vi "Build Field Elements.vi"(10 "Field Half Graph":refnum<vi>, 11 "Field Settings":T1={"Exchange Left"=102.0, "Exchange Right"=150.0, "Power Cube Zone Left"=139.5, "Power Cube Zone Right"=139.5, "Switch Left"=85.25, "Switch Right"=85.25, "Switch Front"=140.0, "Switch Back"=196.0, "Platform Left"=95.25, "Platform Right"=95.25, "Platform Front"=261.47, "Slalom Depth"=235.235}) -> (3 "Field Half":cluster{dbl[], dbl[]}[](graph)=[{[0.0, 36.0, 36.0, 0.0, 0.0], [222.0, 222.0, 174.0, 174.0, 222.0]}, {[101.0, 140.0, 140.0, 101.0, 101.0], [184.5, 184.5, 139.5, 139.5, 184.5]}, {[140.0, 196.0, 196.0, 140.0, 140.0], [238.75, 238.75, 85.25, 85.25, 238.75]}, {[196.0, 209.0, 209.0, 196.0, 196.0], [85.25, 85.25, 98.25, 98.25, 85.25]}, {[196.0, 209.0, 209.0, 196.0, 196.0], [113.35, 113.35, 126.35, 126.35, 113.35]}, {[196.0, 209.0, 209.0, 196.0, 196.0], [141.45, 141.45, 154.45, 154.45, 141.45]}, {[196.0, 209.0, 209.0, 196.0, 196.0], [169.55, 169.55, 182.55, 182.55, 169.55]}, {[196.0, 209.0, 209.0, 196.0, 196.0], [197.65, 197.65, 210.65, 210.65, 197.65]}, {[196.0, 209.0, 209.0, 196.0, 196.0], [225.75, 225.75, 238.75, 238.75, 225.75]}, {[261.47, 386.0, 386.0, 261.47, 261.47], [228.75, 228.75, 95.25, 95.25, 228.75]}])   [LabVIEW 2017]
uses:
  Typedef/Field Settings.ctl
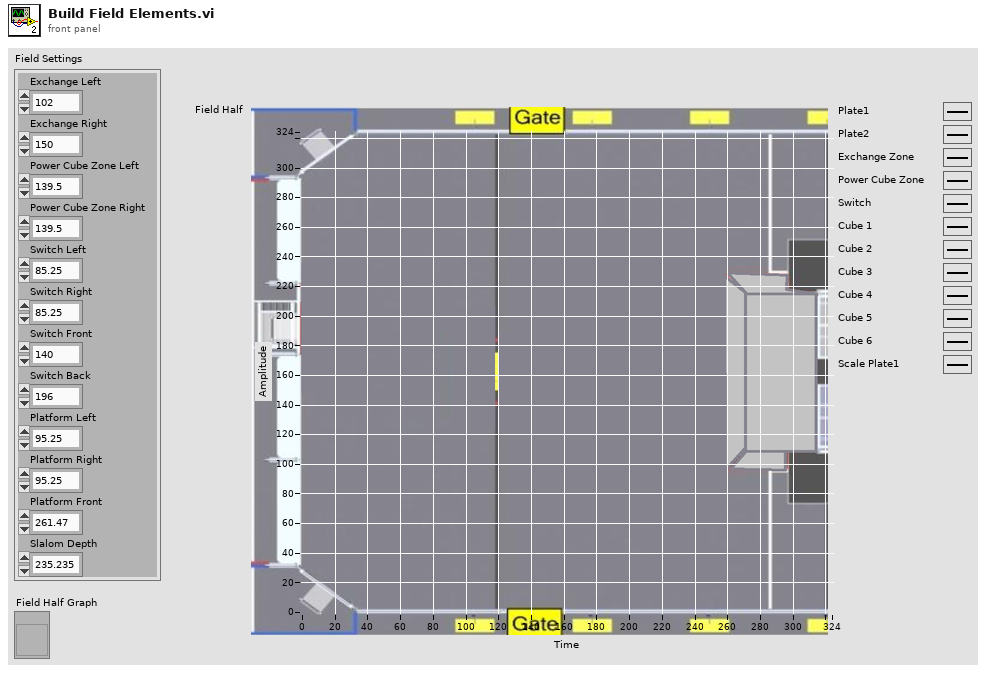
[diagram p1: front panel]
types:
  T1 = typedef "Field Settings.ctl" = cluster{"Exchange Left":dbl, "Exchange Right":dbl, "Power Cube Zone Left":dbl, "Power Cube Zone Right":dbl, "Switch Left":dbl, "Switch Right":dbl, "Switch Front":dbl, "Switch Back":dbl, "Platform Left":dbl, "Platform Right":dbl, "Platform Front":dbl, "Slalom Depth":dbl}
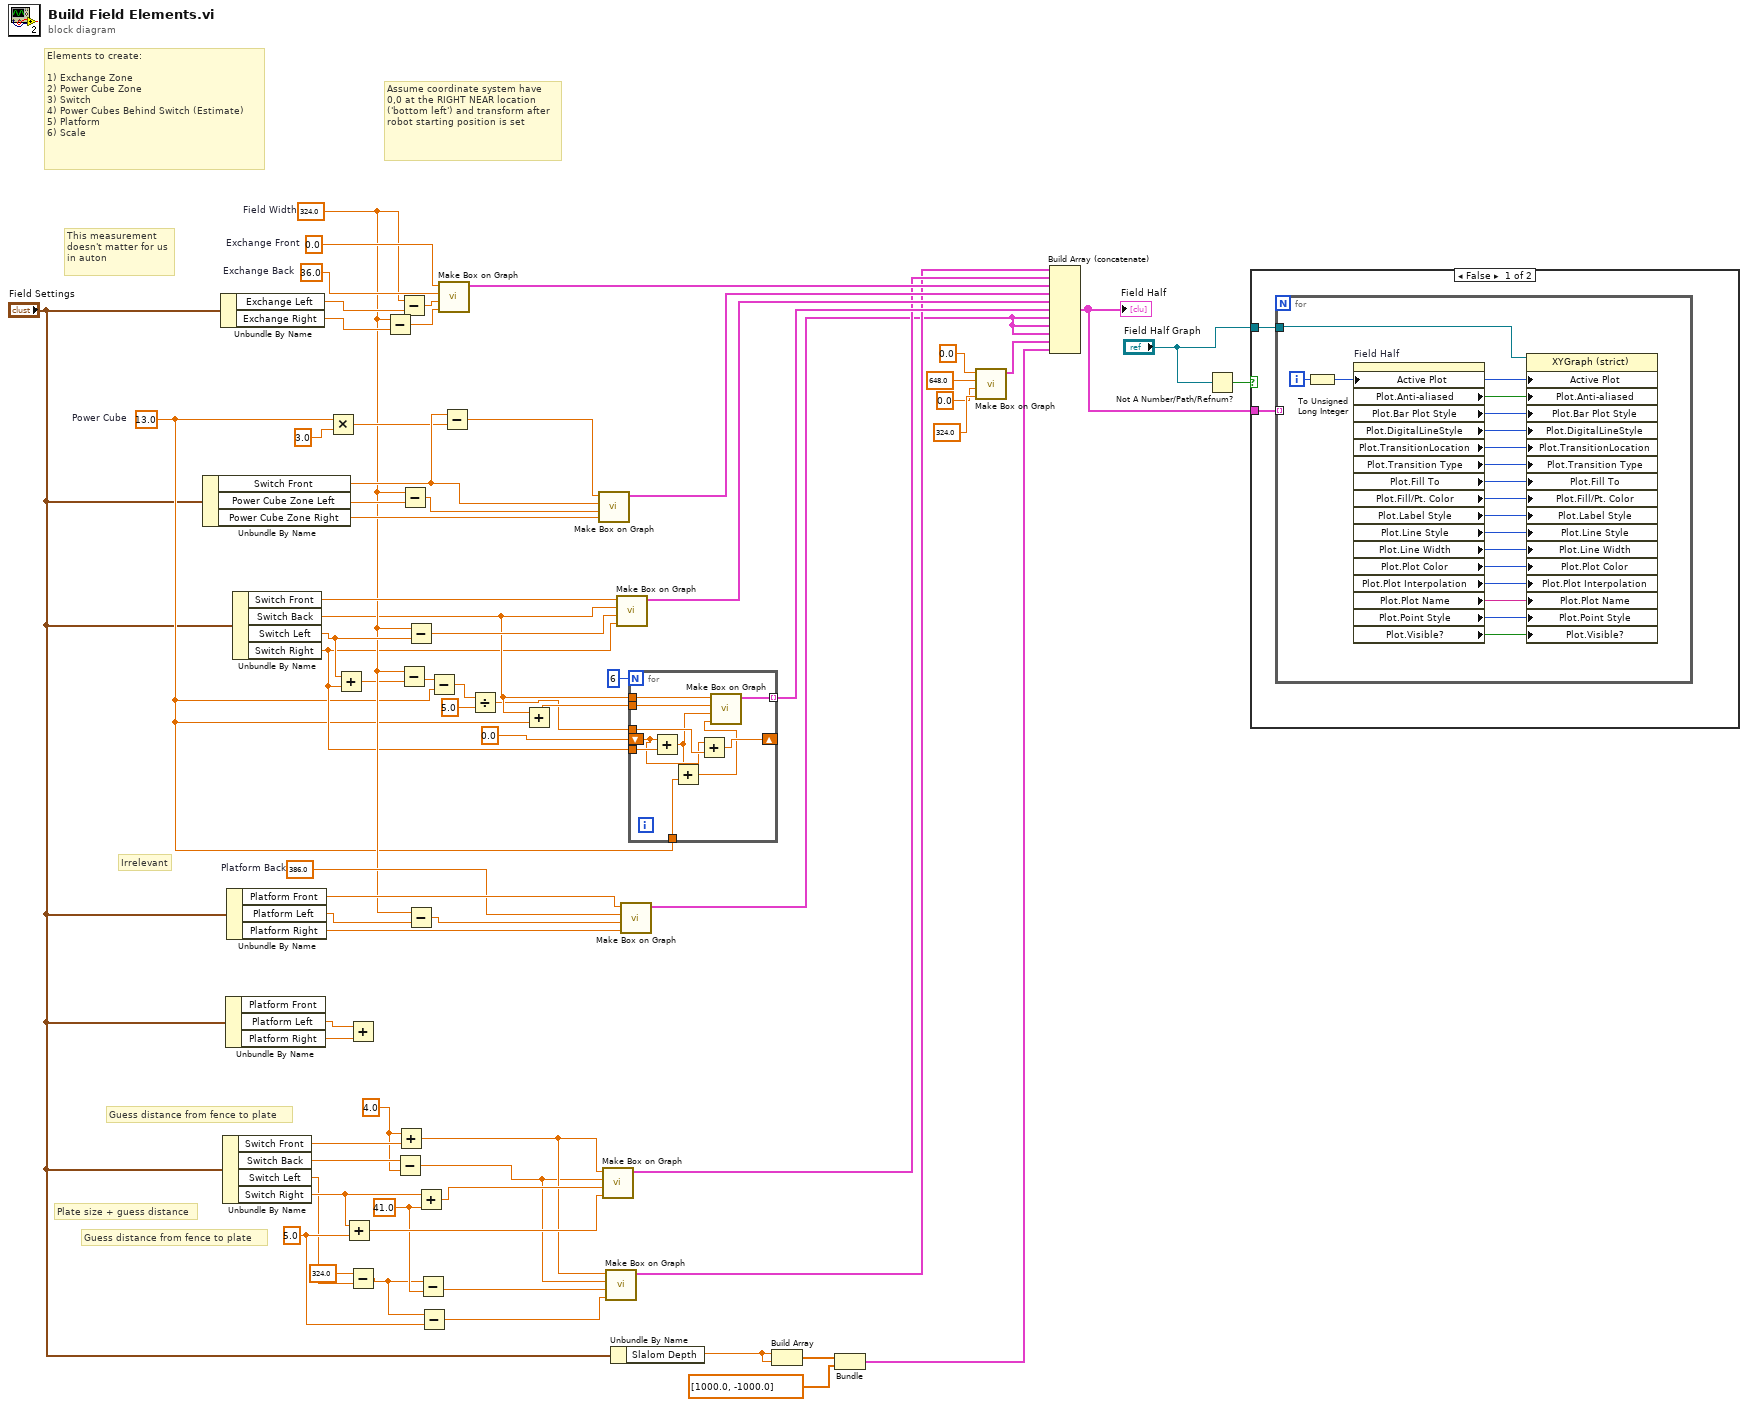
[diagram p0: block diagram]
diagram:
  w19 = 41.0 ("y")
  w17 = 5.0 ("x")
  w26 = 4.0 ("y")
  w49 = 386.0  # Platform Back
  w36 = 13.0  # Power Cube
  w46 = 324.0  # Field Width
  w70 = 36.0  # Exchange Back
  w69 = 0.0  # Exchange Front
  # "Plate size + guess distance"
  # "Guess distance from fence to plate"
  # "Guess distance from fence to plate"
  # "Irrelevant"
  # "Assume coordinate system have 0,0 at the RIGHT NEAR location ('bottom left') and transform after robot starting position is set"
  # "This measurement doesn't matter for us in auton"
  # "Elements to create:\n\n1) Exchange Zone\n2) Power Cube Zone\n3) Switch\n4) Power Cubes Behind Switch (Estimate)\n5) Platform\n6) Scale"
  n1 = Unbundle By Name("Field Settings") -> ("Switch Front"=w59:dbl, "Power Cube Zone Left"=w63:dbl, "Power Cube Zone Right"=w64:dbl)
  n2 = Unbundle By Name("Field Settings") -> ("Exchange Left"=w65:dbl, "Exchange Right"=w68:dbl)
  n3 = Unbundle By Name("Field Settings") -> ("Switch Front"=w28:dbl, "Switch Back"=w27:dbl, "Switch Left"=w14:dbl, "Switch Right"=w25:dbl)
  n4 = Unbundle By Name("Field Settings") -> ("Platform Left"=w31:dbl, "Platform Right"=w30:dbl)  [unwired: 1 out]
  n5 = Unbundle By Name("Field Settings") -> ("Platform Front"=w50:dbl, "Platform Left"=w52:dbl, "Platform Right"=w53:dbl)
  n6 = Unbundle By Name("Field Settings") -> ("Switch Front"=w56:dbl, "Switch Back"=w41:dbl, "Switch Left"=w47:dbl, "Switch Right"=w37:dbl)
  n7 = Multiply(x=w36, y=3.0) -> (x*y=w58:dbl)
  n8 = Add(x=w47, y=w37) -> (x+y=w45:dbl)
  n9 = Add(x=w25, y=w17) -> (x+y=w23:dbl)
  n10 = Add(x=w31, y=w30) -> ()  [unwired: 1 out]
  n11 = Subtract(x=324.0, y=w14) -> (x-y=w13:dbl)
  n12 = Subtract(x=w46, y=w68) -> (x-y=w67:dbl)
  n13 = Subtract(x=w27, y=w26) -> (x-y=w20:dbl)
  n14 = Add(x=w26, y=w28) -> (x+y=w21:dbl)
  n15 = Subtract(x=w46, y=w65) -> (x-y=w66:dbl)
  n16 = Subtract(x=w46, y=w45) -> (x-y=w44:dbl)
  n17 = Subtract(x=w46, y=w63) -> (x-y=w62:dbl)
  n18 = Subtract(x=w46, y=w47) -> (x-y=w55:dbl)
  n19 = Subtract(x=w46, y=w52) -> (x-y=w51:dbl)
  n20 = Add(x=w25, y=w19) -> (x+y=w24:dbl)
  n21 = Subtract(x=w13, y=w19) -> (x-y=w18:dbl)
  n22 = Subtract(x=w13, y=w17) -> (x-y=w16:dbl)
  n23 = Subtract(x=w44, y=w36) -> (x-y=w43:dbl)
  n24 = call "Make Box on Graph.vi"("Y2"=w67, "Y1"=w66, "X2"=w70, "X1"=w69) -> ("Output Graph"=w29:cluster{dbl[], dbl[]})  [unwired: 7 in]
  n25 = Subtract(x=w59, y=w58) -> (x-y=w60:dbl)
  n26 = Divide(x=w43, y=5.0) -> (x/y=w39:dbl)
  n27 = Add(x=w41, y=w36) -> (x+y=w42:dbl)
  n28 = call "Make Box on Graph.vi"("Y2"=w64, "Y1"=w62, "X2"=w59, "X1"=w60) -> ("Output Graph"=w57:cluster{dbl[], dbl[]})  [unwired: 7 in]
  n29 = call "Make Box on Graph.vi"("Y2"=w23, "Y1"=w24, "X2"=w20, "X1"=w21) -> ("Output Graph"=w22:cluster{dbl[], dbl[]})  [unwired: 7 in]
  n30 = call "Make Box on Graph.vi"("Y2"=w16, "Y1"=w18, "X2"=w20, "X1"=w21) -> ("Output Graph"=w15:cluster{dbl[], dbl[]})  [unwired: 7 in]
  n31 = Unbundle By Name("Field Settings") -> ("Slalom Depth"=w4:dbl)
  n32 = call "Make Box on Graph.vi"("Y2"=w37, "Y1"=w55, "X2"=w41, "X1"=w56) -> ("Output Graph"=w54:cluster{dbl[], dbl[]})  [unwired: 7 in]
  n33 = call "Make Box on Graph.vi"("Y2"=w53, "Y1"=w51, "X2"=w49, "X1"=w50) -> ("Output Graph"=w11:cluster{dbl[], dbl[]})  [unwired: 7 in]
  n34 = for {
    N: 6 -> [_]
    tunnel: [w80] -> w48 mode=indexing
    tunnel: w41 -> [w79]
    tunnel: w42 -> [w78]
    tunnel: w39 -> [w77]
    tunnel: w37 -> [w76]
    shift-right: [w75] -> _
    shift-left: 0.0 ("y") -> [w74]
    tunnel: w36 -> [w72]
    n35 = Add(x=w74, y=w76) -> (x+y=w73:dbl)
    n36 = Add(x=w73, y=w72) -> (x+y=w71:dbl)
    n37 = Add(x=w74, y=w77) -> (x+y=w75:dbl)
    n38 = call "Make Box on Graph.vi"("Y2"=w71, "Y1"=w73, "X2"=w78, "X1"=w79) -> ("Output Graph"=w80:cluster{dbl[], dbl[]})  [unwired: 7 in]
  }
  n39 = Build Array(w4, w4) -> (w2:dbl[])
  n40 = Bundle(w2, dbl[] [1000.0, -1000.0]) -> (w1:cluster{dbl[], dbl[]})  [unwired: 1 in]
  n41 = call "Make Box on Graph.vi"("Y2"=324.0, "Y1"=0.0, "X2"=648.0, "X1"=0.0) -> ("Output Graph"=w10:cluster{dbl[], dbl[]})  [unwired: 7 in]
  n42 = Build Array (concatenate)(w15, w22, w29, w57, w54, w48, w11, w11, w11, w10, w1) -> (w34:cluster{dbl[], dbl[]}[])
  "Field Half" <- w34
  n43 = Not A Number/Path/Refnum?(number/path/refnum="Field Half Graph") -> (NaN/Path/Refnum?=w32:bool)
  n44 = case shown="False" w32 {
    tunnel: w34 -> [w82 _]
    tunnel: "Field Half Graph" -> [w81 _]
    frame False {
      n45 = for {
        tunnel: w82 -> [_] mode=indexing
        tunnel: w81 -> [w84]
        i -> [w85]
        n46 = To Unsigned Long Integer(number=w85) -> (unsigned 32bit integer=w83:u32)
        n47 = property on="Field Half" class="XYGraph (strict)"("Active Plot"=w83) -> ("Plot.Anti-aliased"=w100:bool, "Plot.Bar Plot Style"=w99:u8, "Plot.DigitalLineStyle"=w98:u8, "Plot.TransitionLocation"=w97:u8, "Plot.Transition Type"=w96:u8, "Plot.Fill To"=w95:i16, "Plot.Fill/Pt. Color"=w94:u32, "Plot.Label Style"=w93:u8, "Plot.Line Style"=w92:u8, "Plot.Line Width"=w91:u8, "Plot.Plot Color"=w90:u32, "Plot.Plot Interpolation"=w89:u8, "Plot.Plot Name"=w88:string, "Plot.Point Style"=w87:u8, "Plot.Visible?"=w86:bool)  [unwired: 2 in, 2 out]
        n48 = property class="XYGraph (strict)"(reference=w84, "Active Plot"=w83, "Plot.Anti-aliased"=w100, "Plot.Bar Plot Style"=w99, "Plot.DigitalLineStyle"=w98, "Plot.TransitionLocation"=w97, "Plot.Transition Type"=w96, "Plot.Fill To"=w95, "Plot.Fill/Pt. Color"=w94, "Plot.Label Style"=w93, "Plot.Line Style"=w92, "Plot.Line Width"=w91, "Plot.Plot Color"=w90, "Plot.Plot Interpolation"=w89, "Plot.Plot Name"=w88, "Plot.Point Style"=w87, "Plot.Visible?"=w86) -> ()  [unwired: 1 in, 2 out]
      }
    }
    frame True {
    }
  }
